vi "Highlight Bookmark.vi"(8 "Error In":errorcluster, 10 "Data":variant, 11 "State In":T1) -> (0 "Error Out":errorcluster, 3 "State Out":T1)   [LabVIEW 2017, in "Bookmark Manager.lvlib"]
uses:
  Bookmark Manager.lvlib
  Controls/State.ctl
  Controls/VI Bookmark.ctl
  Controls/VI Information.ctl
  Controls/Application Information.ctl
  Controls/Bookmarks Views.ctl
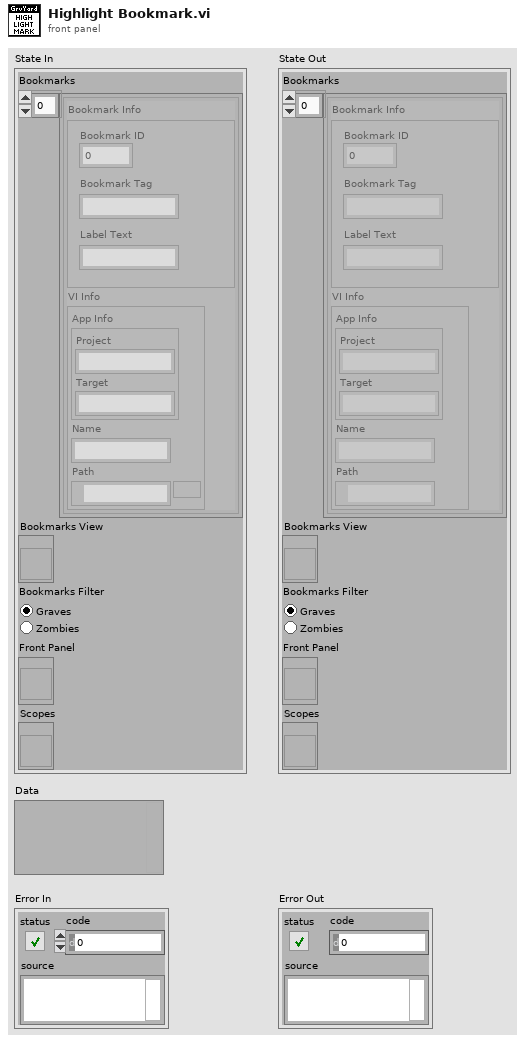
[diagram p1: front panel]
types:
  T1 = typedef "Bookmark Manager.lvlib/State.ctl" = cluster{"Bookmarks":T2[], "Bookmarks View":refnum<vi>, "Bookmarks Filter":T5, "Front Panel":refnum<vi>, "Scopes":refnum<vi>}
  T2 = typedef "Bookmark Manager.lvlib/VI Bookmark.ctl" = cluster{"Bookmark Info":cluster{"Bookmark ID":u32, "Bookmark Tag":string, "Label Text":string}, "VI Info":T3}
  T3 = typedef "Bookmark Manager.lvlib/VI Information.ctl" = cluster{"App Info":T4, "Name":string, "Path":path}
  T4 = typedef "Bookmark Manager.lvlib/Application Information.ctl" = cluster{"Project":string, "Target":string}
  T5 = typedef "Bookmark Manager.lvlib/Bookmarks Views.ctl" = enum32{"Graves", "Zombies"}
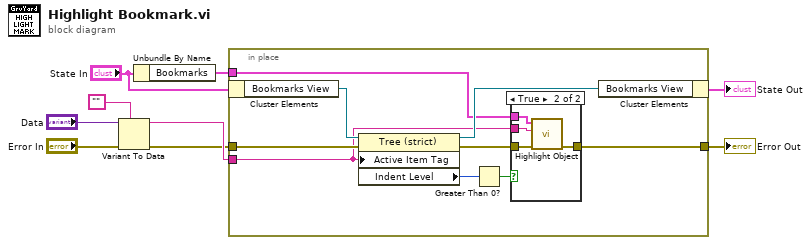
[diagram p0: block diagram]
diagram:
  n1 = Variant To Data(error in="Error In", type="", Variant="Data") -> (data=w7:string, error out=w5:errorcluster)
  n2 = Unbundle By Name("State In") -> ("Bookmarks"=w9:T2[])
  n3 = in-place {
    in-place-border: w5 -> [w16]
    in-place-border: [w12] -> w6
    in-place-border: w7 -> [w10]
    in-place-border: w9 -> [w11]
    n4 = in-place-cluster #1("State In") -> ("Bookmarks View"=w18:refnum<vi>)
    n5 = property class="Tree (strict)"(reference=w18, error in=w16, "Active Item Tag"=w10) -> (reference out=w17:refnum<vi>, error out=w13:errorcluster, "Indent Level"=w15:i32)
    n6 = Greater Than 0?(x=w15) -> (x > 0?=w14:bool)
    n7 = case shown="True" w14 {
      tunnel: w13 -> [w19 w22]
      tunnel: [w19 w21] -> w12
      tunnel: w11 -> [_ w23]
      tunnel: w10 -> [_ w20]
      frame False {
      }
      frame True {
        n8 = call "Highlight Object.vi"("Error In"=w22, "Tag"=w20, "Bookmarks"=w23) -> ("Error Out"=w21:errorcluster)  [unwired: 8 in]
      }
    }
    n9 = in-place-cluster #1("Bookmarks View"=w17) -> (→"State Out":T1)
  }
  "Error Out" <- w6
